vi "JSON String to Variant.vi"(0 "JSON String":string, 7 "Top-Level Control Name":string, 11 "error in (no error)":errorcluster) -> (4 "Variant out":variant, 15 "error out":errorcluster)   [LabVIEW 2017, in "Advanced Variant Tools.lvlib"]
doc: "Unflattens the given JSON string to a JSON instance"
uses:
  Advanced Variant Tools.lvlib
  <vilib>/National Instruments/Variant Data Manipulation/Variant Data Manipulation.lvlib
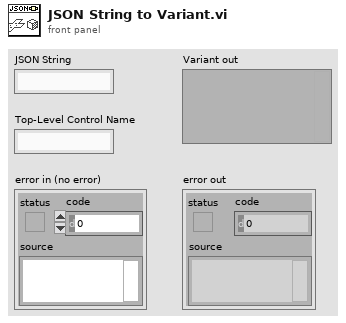
[diagram p1: front panel]
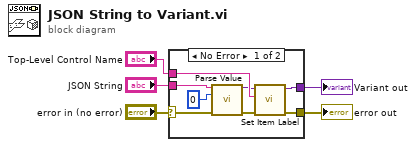
[diagram p0: block diagram]
diagram:
  n1 = case shown="No Error" "error in (no error)" {
    selector: "error in (no error)" -> [w13 w14]
    tunnel: "JSON String" -> [w12 _]
    tunnel: "Top-Level Control Name" -> [w9 _]
    tunnel: [w7 w14] -> w2
    tunnel: [w6 _] -> w1
    frame No Error {
      n2 = call "Parse Value.vi"("JSON String"=w12, "Index In"=0, "error in (no error)"=w13) -> ("Variant out"=w8:variant, "error out"=w10:errorcluster)  [unwired: 10 in, 1 out]
      n3 = call <vilib>:"Set Item Label.vi"("error in (no error)"=w10, "Name"=w9, "Variant in"=w8) -> ("error out"=w7:errorcluster, "Variant out"=w6:variant)  [unwired: 7 in]
    }
    frame Error {
    }
  }
  "error out" <- w2
  "Variant out" <- w1
